vi "quote and escape json string 2.vi"(11 "base string":string) -> (3 "String out":string)   [LabVIEW 2019, in "JSONtext.lvlib"]
uses:
  JSONtext.lvlib
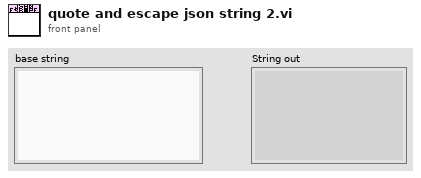
[diagram p1: front panel]
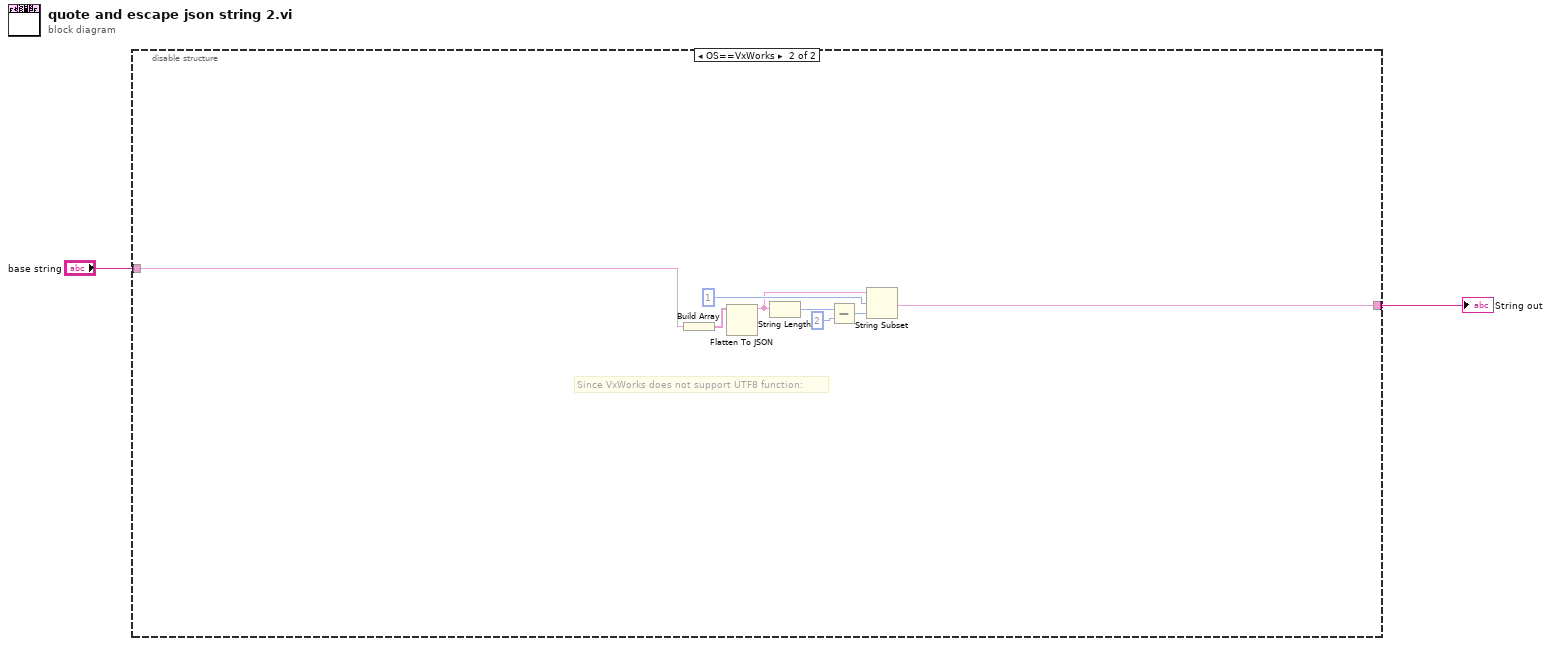
[diagram p0: block diagram]
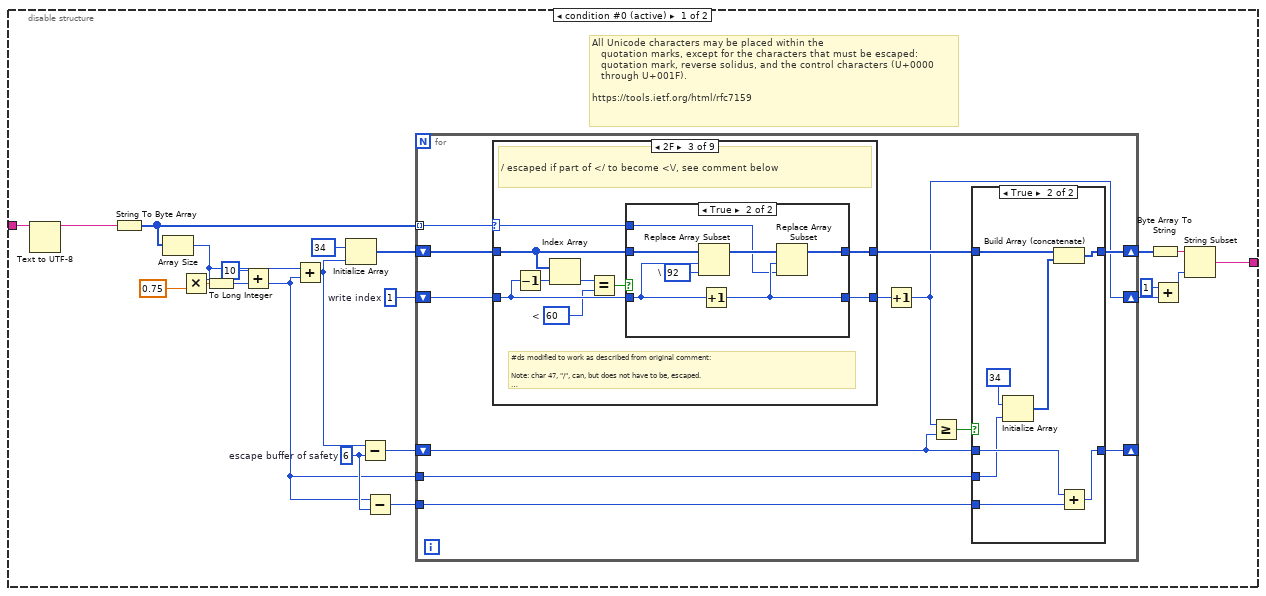
[diagram p2: hidden frame]
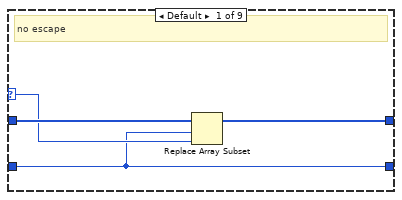
[diagram p4: hidden frame]
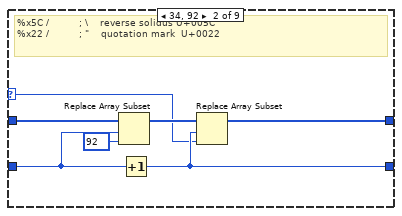
[diagram p5: hidden frame]
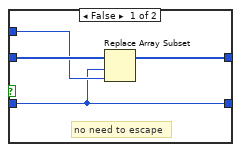
[diagram p6: hidden frame]
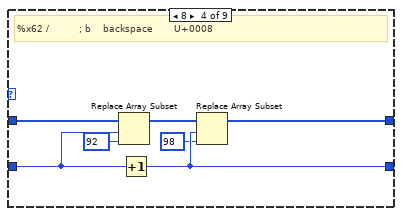
[diagram p7: hidden frame]
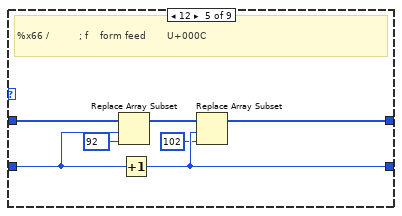
[diagram p8: hidden frame]
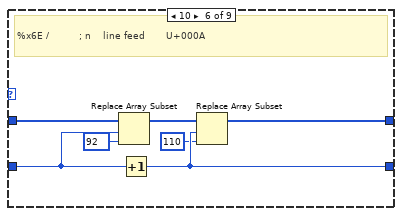
[diagram p9: hidden frame]
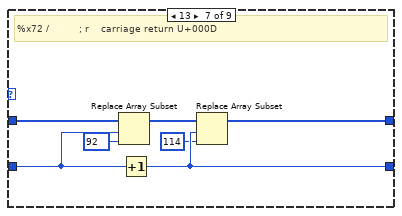
[diagram p10: hidden frame]
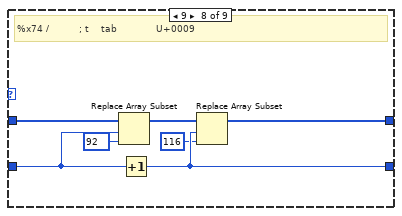
[diagram p11: hidden frame]
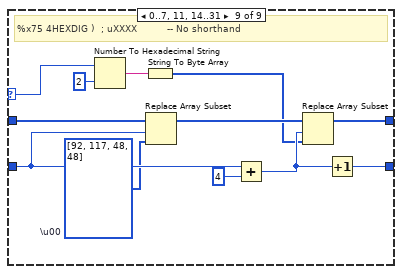
[diagram p12: hidden frame]
diagram:
  n1 = disable-structure shown="OS==VxWorks" {
    disable-tunnel: [w24 w126] -> w2
    disable-tunnel: "base string" -> [w4 w125]
    frame condition #0 (active) {
      w10 = 6  # escape buffer of safety
      w22 = 1  # write index
      # "All Unicode characters may be placed within the\n   quotation marks, except for the characters that must be escaped:\n   quotation mark, reverse solidus, and the control characters (U+0000\n   through U+001F).\n\nhttps://tools.ietf.org/html/rfc7159"
      n2 = Text to UTF-8(11:w4) -> (3:w3:string)  [unwired: 2 in, 1 out]
      n3 = String To Byte Array(string=w3) -> (unsigned byte array=w16:u8[])
      n4 = Array Size(array=w16) -> (size(s)=w14:i32)
      n5 = Multiply(x=w14, y=0.75) -> (x*y=w17:dbl)
      n6 = To Long Integer(number=w17) -> (32bit integer=w11:i32)
      n7 = Add(x=10, y=w11) -> (x+y=w7:i32)
      n8 = Add(x=w14, y=w7) -> (x+y=w13:i32)
      n9 = Initialize Array(u8 34, w13) -> (w19:u8[])
      n10 = Subtract(x=w13, y=w10) -> (x-y=w12:i32)
      n11 = Subtract(x=w7, y=w10) -> (x-y=w9:i32)
      n12 = for {
        shift-right: [w33] -> w21
        shift-left: w19 -> [w36]
        shift-right: [w26] -> w15
        shift-left: w22 -> [w35]
        tunnel: w16 -> [w34] mode=indexing
        shift-right: [w30] -> _
        shift-left: w12 -> [w29]
        tunnel: w7 -> [w28]
        tunnel: w9 -> [w27]
        n13 = case shown="2F" w34 {
          selector: w34 -> [w48 w52 w64 _ _ _ _ _ w121]
          tunnel: w36 -> [w50 w57 w63 w84 w91 w98 w105 w112 w124]
          tunnel: [w49 w54 w66 w81 w88 w95 w102 w109 w123] -> w32
          tunnel: w35 -> [w47 w55 w62 w82 w89 w96 w103 w110 w122]
          tunnel: [w47 w53 w65 w80 w87 w94 w101 w108 w113] -> w31
          frame Default {
            # "no escape"
            n14 = Replace Array Subset(array=w50, new element=w48, index=w47) -> (w49:u8[])
          }
          frame 34, 92 {
            # "%x5C /          ; \\    reverse solidus U+005C\n%x22 /          ; \"    quotation mark  U+0022"
            n15 = Replace Array Subset(array=w57, new element=u8 92 ("new element/subarray"), index=w55) -> (w56:u8[])
            n16 = Increment(x=w55) -> (x+1=w53:i32)
            n17 = Replace Array Subset(array=w56, new element=w52, index=w53) -> (w54:u8[])
          }
          frame 47 {
            w58 = u8 60  # <
            # "#ds modified to work as described from original comment:\n\nNote: char 47, \"/\", can, but does not have to be, escaped.\n\nSee Errata 3159 for RFC4627.   -- JDP\n\nSo we only escape \"/\" if it is part of \"</\", as this is\nthe case that needs escaping to put JSON in a\n<script>...</script> HTML tag  -- JDP Nov, 2014"
            # "/ escaped if part of </ to become <\\/, see comment below"
            n18 = Decrement(x=w62) -> (x-1=w61:i32)
            n19 = Index Array(array=w63, index=w61) -> (element=w60:u8)
            n20 = Equal?(x=w60, y=w58) -> (x = y?=w59:bool)
            n21 = case shown="True" w59 {
              tunnel: [w69 w76] -> w66
              tunnel: [w67 w75] -> w65
              tunnel: w64 -> [w68 w74]
              tunnel: w63 -> [w70 w73]
              tunnel: w62 -> [w67 w72]
              frame False {
                # "no need to escape"
                n22 = Replace Array Subset(array=w70, new element=w68, index=w67) -> (w69:u8[])
              }
              frame True {
                w71 = u8 92  # \
                n23 = Replace Array Subset(array=w73, new element=w71, index=w72) -> (w77:u8[])
                n24 = Increment(x=w72) -> (x+1=w75:i32)
                n25 = Replace Array Subset(array=w77, new element=w74, index=w75) -> (w76:u8[])
              }
            }
          }
          frame 8 {
            # "%x62 /          ; b    backspace       U+0008"
            n26 = Replace Array Subset(array=w84, new element=u8 92 ("new element/subarray"), index=w82) -> (w83:u8[])
            n27 = Increment(x=w82) -> (x+1=w80:i32)
            n28 = Replace Array Subset(array=w83, new element=u8 98 ("new element/subarray"), index=w80) -> (w81:u8[])
          }
          frame 12 {
            # "%x66 /          ; f    form feed       U+000C"
            n29 = Replace Array Subset(array=w91, new element=u8 92 ("new element/subarray"), index=w89) -> (w90:u8[])
            n30 = Increment(x=w89) -> (x+1=w87:i32)
            n31 = Replace Array Subset(array=w90, new element=u8 102 ("new element/subarray"), index=w87) -> (w88:u8[])
          }
          frame 10 {
            # "%x6E /          ; n    line feed       U+000A"
            n32 = Replace Array Subset(array=w98, new element=u8 92 ("new element/subarray"), index=w96) -> (w97:u8[])
            n33 = Increment(x=w96) -> (x+1=w94:i32)
            n34 = Replace Array Subset(array=w97, new element=u8 110 ("new element/subarray"), index=w94) -> (w95:u8[])
          }
          frame 13 {
            # "%x72 /          ; r    carriage return U+000D"
            n35 = Replace Array Subset(array=w105, new element=u8 92 ("new element/subarray"), index=w103) -> (w104:u8[])
            n36 = Increment(x=w103) -> (x+1=w101:i32)
            n37 = Replace Array Subset(array=w104, new element=u8 114 ("new element/subarray"), index=w101) -> (w102:u8[])
          }
          frame 9 {
            # "%x74 /          ; t    tab             U+0009"
            n38 = Replace Array Subset(array=w112, new element=u8 92 ("new element/subarray"), index=w110) -> (w111:u8[])
            n39 = Increment(x=w110) -> (x+1=w108:i32)
            n40 = Replace Array Subset(array=w111, new element=u8 116 ("new element/subarray"), index=w108) -> (w109:u8[])
          }
          frame 0..7, 11, 14..31 {
            w114 = u8[] [92, 117, 48, 48]  # \u00
            # "%x75 4HEXDIG )  ; uXXXX          -- No shorthand"
            n41 = Number To Hexadecimal String(1:i16 2 ("width (-)"), 2:w121) -> (0:w116:string)
            n42 = String To Byte Array(string=w116) -> (unsigned byte array=w118:u8[])
            n43 = Replace Array Subset(array=w124, new element=w114, index=w122) -> (w120:u8[])
            n44 = Add(x=w122, y=4) -> (x+y=w119:i32)
            n45 = Replace Array Subset(array=w120, new element=w118, index=w119) -> (w123:u8[])
            n46 = Increment(x=w119) -> (x+1=w113:i32)
          }
        }
        n47 = Increment(x=w31) -> (x+1=w26:i32)
        n48 = Greater Or Equal?(x=w26, y=w29) -> (x >= y?=w25:bool)
        n49 = case shown="True" w25 {
          tunnel: [w38 w41] -> w33
          tunnel: w32 -> [w38 w42]
          tunnel: [w37 w44] -> w30
          tunnel: w29 -> [w37 w45]
          tunnel: w28 -> [_ w43]
          tunnel: w27 -> [_ w46]
          frame False {
          }
          frame True {
            n50 = Initialize Array(u8 34, w43) -> (w40:u8[])
            n51 = Build Array (concatenate)(w42, w40) -> (w41:u8[])
            n52 = Add(x=w45, y=w46) -> (x+y=w44:i32)
          }
        }
      }
      n53 = Byte Array To String(unsigned byte array=w21) -> (string=w23:string)
      n54 = Add(x=1, y=w15) -> (x+y=w8:i32)
      n55 = String Subset(string=w23, length (rest)=w8) -> (substring=w24:string)  [unwired: 1 in]
    }
    frame condition #1 {
      # "Since VxWorks does not support UTF8 function:"
      n56 = Build Array(w125) -> (w132:string[])
      n57 = Flatten To JSON(anything=w132) -> (JSON string=w129:string)  [unwired: 2 in, 1 out]
      n58 = String Length(string=w129) -> (length=w130:i32)
      n59 = Subtract(x=w130, y=2 ("x")) -> (x-y=w128:i32)
      n60 = String Subset(string=w129, offset (0)=1, length (rest)=w128) -> (substring=w126:string)
    }
  }
  "String out" <- w2
